vi "read maps dynamically.vi"(8 "error in":errorcluster, 11 "module configuration in":refnum<class "TDMS datalogger configuration.lvclass">) -> (0 "error out":errorcluster, 2 "maps dynamically":bool, 3 "module configuration out":refnum<class "TDMS datalogger configuration.lvclass">)   [LabVIEW 2013, in "TDMS datalogger configuration.lvclass"]
doc: "Provides an interface for determining if a runtime module associated with this configuration is capable of dynamically mapping to channels through <b>dynamic mapping.vi</b>."
uses:
  TDMS datalogger configuration.lvclass
  TDMS datalogger configuration.lvclass/TDMS datalogger configuration.ctl
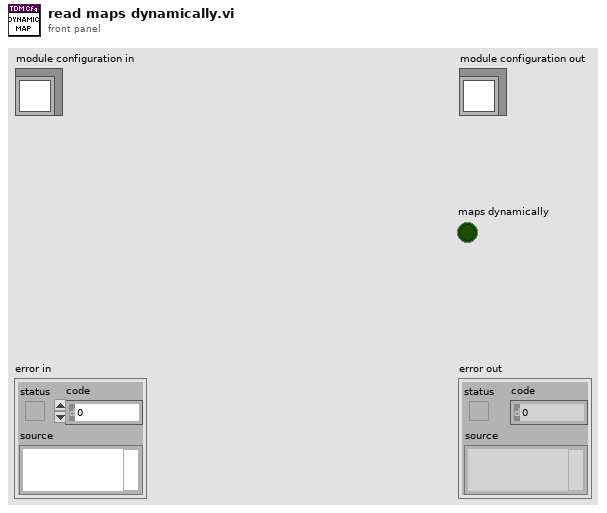
[diagram p1: front panel]
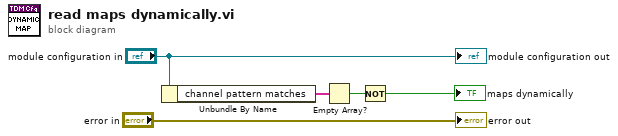
[diagram p0: block diagram]
diagram:
  n1 = Unbundle By Name("module configuration in") -> ("channel pattern matches"=w3:string[])
  n2 = Empty Array?(array=w3) -> (empty?=w2:bool)
  n3 = Not(x=w2) -> (.not. x?=→"maps dynamically":bool)
  "error out" <- "error in"
  "module configuration out" <- "module configuration in"
